vi "create single value wavelength of desired length (length value in).vi"(9 "waveform (with desired single value)":waveform(dbl), 11 "length in":i32) -> (3 "output waveform":waveform(dbl))   [LabVIEW 2025]
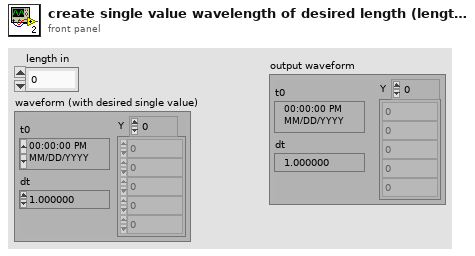
[diagram p1: front panel]
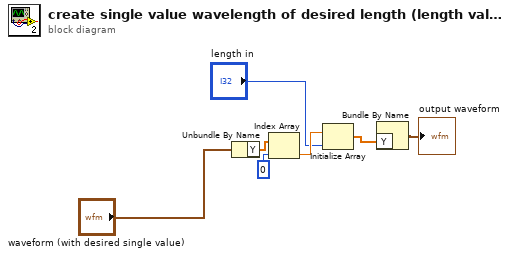
[diagram p0: block diagram]
diagram:
  n1 = Unbundle By Name("waveform (with desired single value)") -> ("Y"=w7:dbl[])
  n2 = Index Array(array=w7, index=0) -> (element=w5:dbl)
  n3 = Initialize Array(w5, "length in") -> (w4:dbl[])
  n4 = Bundle By Name("Y"=w4) -> (→"output waveform":waveform(dbl))  [unwired: 1 in]
